vi "DepthCalibrationTable.vi"(11 "DS5CalibrationCoefficientsTable":u8[](array[numeric])=[21, 0, 0, 0, 3, 0, 25, 0, 240, 1, 0, 0, 0, 4, 0, 4, 169, 238, 63, 236, 156, 141, 55, 63, 113, 190, 162, 63, 135, 142, 252, 62, 9, 233, 5, 63, 31, 150, 10, 62, 55, 118, 207, 190, 113, 68, 102, 58, 249, 138, 146, 186, 37, 191, 183, 62, 140, 183, 56, 63, 9, 210, 163, 63, 166, 65, 2, 63, 224, 139, 1, 63, 100, 118, 2, 62, 234, 150, 203, 190, 17, 251, 198, 57, 162, 214, 21, 187, 174, 168, 180, 62, 233, 255, 127, 63, 123, 123, 122, 58, 169, 40, 178, 186, 91, 254, 122, 186, 231, 255, 127, 63, 249, 16, 188, 186, 151, 250, 177, 58, 148, 60, 188, 58, 223, 255, 127, 63, 253, 254, 127, 63, 187, 169, 2, 187, 133, 7, 170, 187, 170, 38, 3, 59, 205, 255, 127, 63, 195, 120, 187, 58, 120, 239, 169, 59, 115, 212, 188, 186, 13, 255, 127, 63, 197, 83, 91, 194, 1, 0, 0, 0, 0, 0, 0, 0, 0, 0, 0, 0, 0, 0, 0, 0, 0, 0, 0, 0, 0, 0, 0, 0, 0, 0, 0, 0, 0, 0, 0, 0, 0, 0, 0, 0, 0, 0, 0, 0, 0, 0, 0, 0, 0, 0, 0, 0, 0, 0, 0, 0, 0, 0, 0, 0, 0, 0, 0, 0, 0, 0, 0, 0, 0, 0, 0, 0, 0, 0, 0, 0, 0, 0, 0, 0, 0, 0, 0, 0, 0, 0, 0, 0, 0, 0, 0, 0, 0, 0, 0, 0, 27, 157, 178, 68, 27, 157, 178, 68, 254, 246, 109, 68, 45, 3, 11, 68, 207, 38, 110, 68, 207, 38, 110, 68, 169, 164, 30, 68, 145, 89, 185, 67, 138, 196, 30, 68, 138, 196, 30, 68, 225, 48, 158, 67, 23, 34, 119, 67, 138, 196, 30, 68, 138, 196, 30, 68, 225, 48, 210, 67, 23, 34, 119, 67, 207, 38, 238, 67, 207, 38, 238, 67, 169, 164, 158, 67, 145, 89, 57, 67, 138, 196, 158, 67, 138, 196, 158, 67, 225, 48, 82, 67, 23, 34, 247, 66, 138, 196, 158, 67, 138, 196, 158, 67, 225, 48, 30, 67, 23, 34, 247, 66, 27, 157, 178, 67, 27, 157, 178, 67, 254, 246, 109, 67, 45, 3, 11, 67, 115, 78, 132, 68, 115, 78, 132, 68, 17, 126, 30, 68, 190, 241, 205, 67, 27, 157, 50, 68, 27, 157, 50, 68, 254, 246, 237, 67, 45, 3, 139, 67, 0, 0, 0, 0, 0, 0, 0, 0, 0, 0, 0, 0, 0, 0, 0, 0, 0, 0, 0, 0, 0, 0, 0, 0, 0, 0, 0, 0, 0, 0, 0, 0, 0, 0, 0, 0, 0, 0, 0, 0, 0, 0, 0, 0, 0, 0, 0, 0, 0, 0, 0, 0, 0, 0, 0, 0, 0, 0, 0, 0, 0, 0, 0, 0, 0, 0, 0, 0, 0, 0, 0, 0, 0, 0, 0, 0, 0, 0, 0, 0, 0, 0, 0, 0, 0, 0, 0, 0, 0, 0, 0, 0, 0, 0, 0, 0, 0, 0, 0, 0, 105, 207, 27, 52, 0, 14, 0, 128, 67, 0, 58, 0, 92, 0, 80, 0, 114, 0, 111, 0, 103, 0, 114, 0, 97, 0, 109, 0, 32, 0, 70, 0, 105, 0, 108, 0, 101, 0, 115, 0, 92, 0, 78, 0, 97, 0, 116, 0, 105, 0, 111, 0, 110, 0, 97, 0, 108, 0, 32, 0, 73, 0, 110, 0, 115, 0, 116, 0, 114, 0, 117, 0, 109, 0, 101, 0, 110, 0, 116, 0, 115, 0, 92, 0, 76, 0, 97, 0, 98, 0, 86, 0, 73, 0, 69, 0, 87, 0, 32, 0, 50, 0, 48, 0, 49, 0, 54, 0, 92, 0, 76, 0, 97, 0, 98, 0, 86, 0, 73, 0, 69, 0, 87, 0, 46, 0, 101, 0, 120, 0, 101, 0, 0, 0, 114, 0, 101, 0, 92, 0, 112, 0, 110, 0, 103, 0, 46, 0, 108, 0, 108, 0, 98, 0, 0, 0, 0, 0, 0, 0, 0, 0, 0, 0, 0, 0, 0, 0, 0, 0, 0, 0, 0, 0, 0, 0, 0, 0, 0, 0, 0, 0, 0, 0, 0, 0, 0, 0, 0, 0, 0, 0, 0, 0, 0, 0, 0, 0, 0, 0, 0, 0, 0, 0, 0, 0, 0, 0, 0, 0, 0, 0, 0, 0, 0, 0, 0, 0, 0, 0, 0, 0, 0, 0, 0, 0, 0, 0, 0, 0, 0, 0, 0, 0, 0, 0, 0, 0, 0, 0, 0, 0, 0, 0, 0, 0, 0, 0, 0, 0, 0, 0, 0, 0, 0, 0, 0, 0, 0, 0, 0, 0, 0, 0, 0, 0, 0, 0, 0, 0, 0, 0, 0, 0, 0, 0, 0, 0, 0, 0, 0, 0, 0, 0, 0, 0, 0, 0, 0, 0, 0, 0, 0, 0, 0, 0, 0, 0, 0, 0, 0, 0, 0, 0, 0, 0, 0, 0, 0, 0, 0, 0, 0, 0, 0, 0, 0, 0, 0, 0, 0, 0, 0, 0, 0, 0, 0, 0, 0, 0, 0, 0, 0, 0, 0, 0, 0, 0, 0, 0, 0, 0, 0, 0, 0, 0, 0, 0, 0, 0, 0, 0, 0, 0, 0, 0, 0, 0, 0, 0, 0, 0, 0, 0, 0, 0, 0, 0, 0, 0, 0, 0, 0, 0, 0, 0, 0, 0, 0, 0, 0, 0, 0, 0, 0, 0, 0, 0, 0, 0, 0, 0, 0, 0, 0, 0, 0, 0, 0, 0, 0, 0, 0, 0, 0, 0, 0, 0, 0, 0, 0, 0, 0, 0, 0, 0, 0, 0, 0, 0, 0, 0, 0, 0, 0, 0, 0, 0, 0, 0, 0, 0, 0, 0, 0, 0, 0, 0, 0, 0, 0, 0, 0, 0, 0, 0, 0, 0, 0, 0, 0, 0, 0, 0, 0, 0, 0, 0, 0, 0, 0, 0, 0, 0, 0, 0, 0, 0, 0, 0, 0, 0, 0, 0, 0, 0, 0, 0, 0, 0, 0, 0, 0, 0, 0, 0, 0, 0, 0, 0, 0, 0, 0, 0, 0, 0, 0, 0, 0, 0, 0, 0, 0, 0] format="%x") -> (0 "table reserved 2":sgl[](array[numeric])=[714.4548, 714.4548, 475.92963, 278.0248], 1 "table reserved 1":sgl[](array[numeric])=[714.4548, 714.4548, 475.92963, 278.0248], 2 "New Calibration Parameters":T1={"fx"=0.71700454, "fy"=1.2714368, "px"=0.4932749, "py"=0.5230871, "k left"=[0.13533829, -0.40519878, 0.0008784002, -0.0011180333, 0.3588802], "fx2"=0.7215507, "fy2"=1.2798473, "py2"=0.5060406, "px2"=0.5088142, "k right"=[0.12740475, -0.39763576, 0.00037952562, -0.0022863527, 0.35284942], "RLeft"=[0.9999986, 0.0009555143, -0.001359244, -0.0009574645, 0.9999985, -0.001434832, 0.001357871, 0.0014361315, 0.99999803], "Rright"=[0.99998456, -0.0019937593, -0.0051888847, 0.002001206, 0.99999696, 0.0014302958, 0.0051860176, -0.0014406577, 0.9999855], "baseline"=-54.831806, "useBrownModel"=1, "1280x720"=[952.6064, 952.6064, 634.5728, 370.69974]}, 3 "Calibration table":T2={"version"=3, "table type"=60479, "table size"=496, "full version"=67109888, "crc32"=3963612841, "baseline"=-54.831806, "model"=1, "fx left"=917.7658, "fy left"=915.4345, "px left"=631.39185, "py left"=376.6227, "py right"=364.3492, "px right"=651.2822, "fy right"=921.49005, "fx right"=923.5849, "k left"=[0.13533829, -0.40519878, 0.0008784002, -0.0011180333, 0.3588802], "k right"=[0.12740475, -0.39763576, 0.00037952562, -0.0022863527, 0.35284942], "RLeft"=[0.9999986, 0.0009555143, -0.001359244, -0.0009574645, 0.9999985, -0.001434832, 0.001357871, 0.0014361315, 0.99999803], "Rright"=[0.99998456, -0.0019937593, -0.0051888847, 0.002001206, 0.99999696, 0.0014302958, 0.0051860176, -0.0014406577, 0.9999855], "uint8 reserved1"=[0, 0, 0, 0, 0, 0, 0, 0, 0, 0, 0, 0, 0, 0, 0, 0, 0, 0, 0, 0, 0, 0, 0, 0, 0, 0, 0, 0, 0, 0, 0, 0, 0, 0, 0, 0, 0, 0, 0, 0, 0, 0, 0, 0, 0, 0, 0, 0, 0, 0, 0, 0, 0, 0, 0, 0, 0, 0, 0, 0, 0, 0, 0, 0, 0, 0, 0, 0, 0, 0, 0, 0, 0, 0, 0, 0, 0, 0, 0, 0, 0, 0, 0, 0, 0, 0, 0, 0], "uint8 reserved2"=[0, 0, 0, 0, 0, 0, 0, 0, 0, 0, 0, 0, 0, 0, 0, 0, 0, 0, 0, 0, 0, 0, 0, 0, 0, 0, 0, 0, 0, 0, 0, 0, 0, 0, 0, 0, 0, 0, 0, 0, 0, 0, 0, 0, 0, 0, 0, 0, 0, 0, 0, 0, 0, 0, 0, 0, 0, 0, 0, 0, 0, 0, 0, 0], "1920x1080"=[1428.9095, 1428.9095, 951.85925, 556.0496], "1280x720"=[952.6064, 952.6064, 634.5728, 370.69974], "640x480"=[635.0709, 635.0709, 316.38187, 247.13316], "848x480"=[635.0709, 635.0709, 420.38187, 247.13316], "640x360"=[476.3032, 476.3032, 317.2864, 185.34987], "424x240"=[317.53546, 317.53546, 210.19093, 123.56658], "320x240"=[317.53546, 317.53546, 158.19093, 123.56658], "480x270"=[357.2274, 357.2274, 237.96481, 139.0124], "1280x800"=[1058.4515, 1058.4515, 633.9698, 411.8886], "960x540"=[714.4548, 714.4548, 475.92963, 278.0248], "Reserved1"=[714.4548, 714.4548, 475.92963, 278.0248], "Reserved 2"=[714.4548, 714.4548, 475.92963, 278.0248]} {"crc32" format="%x"})   [LabVIEW 2017, in "libRealSense3.lvlib"]
uses:
  libRealSense3.lvlib
panel:
  out "x+y":i32
  out "700":sgl[](array[numeric])=[1428.9095, 1428.9095, 951.85925, 556.0496]
  out "500":sgl[](array[numeric])=[1428.9095, 1428.9095, 951.85925, 556.0496]
  out "uint8 reserved2 2":u8[](array[numeric])
  out "Input size":i32
  out "size(s) 2":i32
  out "size(s)":i32
  out "size":i32
  out "subarray":u8[](array[numeric])=[156, 141, 55, 63, 113, 190, 162, 63, 135, 142, 252, 62, 9, 233, 5, 63, 31, 150, 10, 62, 55, 118, 207, 190, 113, 68, 102, 58, 249, 138, 146, 186, 37, 191, 183, 62] format="%x"
  out "Output array":u8[](array[numeric])=[3, 0, 25, 0, 240, 1, 0, 0, 0, 4, 0, 4, 169, 238, 63, 236, 156, 141, 55, 63, 113, 190, 162, 63, 135, 142, 252, 62, 9, 233, 5, 63, 31, 150, 10, 62, 55, 118, 207, 190, 113, 68, 102, 58, 249, 138, 146, 186, 37, 191, 183, 62, 140, 183, 56, 63, 9, 210, 163, 63, 166, 65, 2, 63, 224, 139, 1, 63, 100, 118, 2, 62, 234, 150, 203, 190, 17, 251, 198, 57, 162, 214, 21, 187, 174, 168, 180, 62, 233, 255, 127, 63, 123, 123, 122, 58, 169, 40, 178, 186, 91, 254, 122, 186, 231, 255, 127, 63, 249, 16, 188, 186, 151, 250, 177, 58, 148, 60, 188, 58, 223, 255, 127, 63, 253, 254, 127, 63, 187, 169, 2, 187, 133, 7, 170, 187, 170, 38, 3, 59, 205, 255, 127, 63, 195, 120, 187, 58, 120, 239, 169, 59, 115, 212, 188, 186, 13, 255, 127, 63, 197, 83, 91, 194, 1, 0, 0, 0, 0, 0, 0, 0, 0, 0, 0, 0, 0, 0, 0, 0, 0, 0, 0, 0, 0, 0, 0, 0, 0, 0, 0, 0, 0, 0, 0, 0, 0, 0, 0, 0, 0, 0, 0, 0, 0, 0, 0, 0, 0, 0, 0, 0, 0, 0, 0, 0, 0, 0, 0, 0, 0, 0, 0, 0, 0, 0, 0, 0, 0, 0, 0, 0, 0, 0, 0, 0, 0, 0, 0, 0, 0, 0, 0, 0, 0, 0, 0, 0, 0, 0, 0, 0, 0, 0, 0, 0, 27, 157, 178, 68, 27, 157, 178, 68, 254, 246, 109, 68, 45, 3, 11, 68, 207, 38, 110, 68, 207, 38, 110, 68, 169, 164, 30, 68, 145, 89, 185, 67, 138, 196, 30, 68, 138, 196, 30, 68, 225, 48, 158, 67, 23, 34, 119, 67, 138, 196, 30, 68, 138, 196, 30, 68, 225, 48, 210, 67, 23, 34, 119, 67, 207, 38, 238, 67, 207, 38, 238, 67, 169, 164, 158, 67, 145, 89, 57, 67, 138, 196, 158, 67, 138, 196, 158, 67, 225, 48, 82, 67, 23, 34, 247, 66, 138, 196, 158, 67, 138, 196, 158, 67, 225, 48, 30, 67, 23, 34, 247, 66, 27, 157, 178, 67, 27, 157, 178, 67, 254, 246, 109, 67, 45, 3, 11, 67, 115, 78, 132, 68, 115, 78, 132, 68, 17, 126, 30, 68, 190, 241, 205, 67, 27, 157, 50, 68, 27, 157, 50, 68, 254, 246, 237, 67, 45, 3, 139, 67] format="%x"
  out "Baseline":u8[](array[numeric])=[194, 91, 83, 197]
  out "reversed array":u8[](array[numeric])=[194, 91, 83, 197]
  out "960x540":sgl[](array[numeric])=[714.4548, 714.4548, 475.92963, 278.0248]
  out "1280x800":sgl[](array[numeric])=[1058.4515, 1058.4515, 633.9698, 411.8886]
  out "480x270":sgl[](array[numeric])=[357.2274, 357.2274, 237.96481, 139.0124]
  out "320x240":sgl[](array[numeric])=[317.53546, 317.53546, 158.19093, 123.56658]
  out "424x240":sgl[](array[numeric])=[317.53546, 317.53546, 210.19093, 123.56658]
  out "640x360":sgl[](array[numeric])=[476.3032, 476.3032, 317.2864, 185.34987]
  out "848x480":sgl[](array[numeric])=[635.0709, 635.0709, 420.38187, 247.13316]
  out "640x480":sgl[](array[numeric])=[635.0709, 635.0709, 316.38187, 247.13316]
  out "1280x720":sgl[](array[numeric])=[952.6064, 952.6064, 634.5728, 370.69974]
  out "1920x1080":sgl[](array[numeric])=[1428.9095, 1428.9095, 951.85925, 556.0496]
  out "uint8 reserved2":u8[](array[numeric])
  out "uint8 reserved1":u8[](array[numeric])
  out "model":u32=1
  out "baseline":sgl=-54.831806
  out "Rright":sgl[](array[numeric])=[0.99998456, -0.0019937593, -0.0051888847, 0.002001206, 0.99999696, 0.0014302958, 0.0051860176, -0.0014406577, 0.9999855]
  out "RLeft":sgl[](array[numeric])=[0.9999986, 0.0009555143, -0.001359244, -0.0009574645, 0.9999985, -0.001434832, 0.001357871, 0.0014361315, 0.99999803]
  out "crc32":u32=3963612841
  out "full version":u32=67109888
  out "table size":u32=496
  out "table type":u16=25
  out "version":u16=3
  out "fx2":sgl=0.7215507
  out "fy2":sgl=1.2798473
  out "px2":sgl=0.5088142
  out "py2":sgl=0.5060406
  out "k right":sgl[](array[numeric])=[0.12740475, -0.39763576, 0.00037952562, -0.0022863527, 0.35284942]
  out "k left":sgl[](array[numeric])=[0.13533829, -0.40519878, 0.0008784002, -0.0011180333, 0.3588802]
  out "py":sgl=0.5230871
  out "px":sgl=0.4932749
  out "fy":sgl=1.2714368
  out "fx":sgl=0.71700454
  # "this is to get coefficents"
  # "//! DS5 calibration coefficients table. Table ID is 0x19.\nstruct DS5CalibrationCoefficientsTable\n{\n\tDS5CalibrationTableHeader header;       //!< Header\n\tDS5CalibrationCoefficients coeffs;      //!< Coefficients\n\tDS5CoeffsMode  modes[12];               //!< Rectified camera parameters. Each entry in the table corresponds to a resolution\n\tuint8_t  reserved2[64];                 //!< Reserved\n};"
  # "Use this one to set through intermediate"
  # "//! Structure used to update the calibration during live streaming using the CALIBRECALC command\nstruct DS5CalibrationCoefficientsUpdateParam\n{\n\tDS5CalibrationCoefficients coeffs;      //!< Coefficients\n\tDS5CoeffsMode mode;                     //!< Rectified camera parameters for the current resolution\n};"
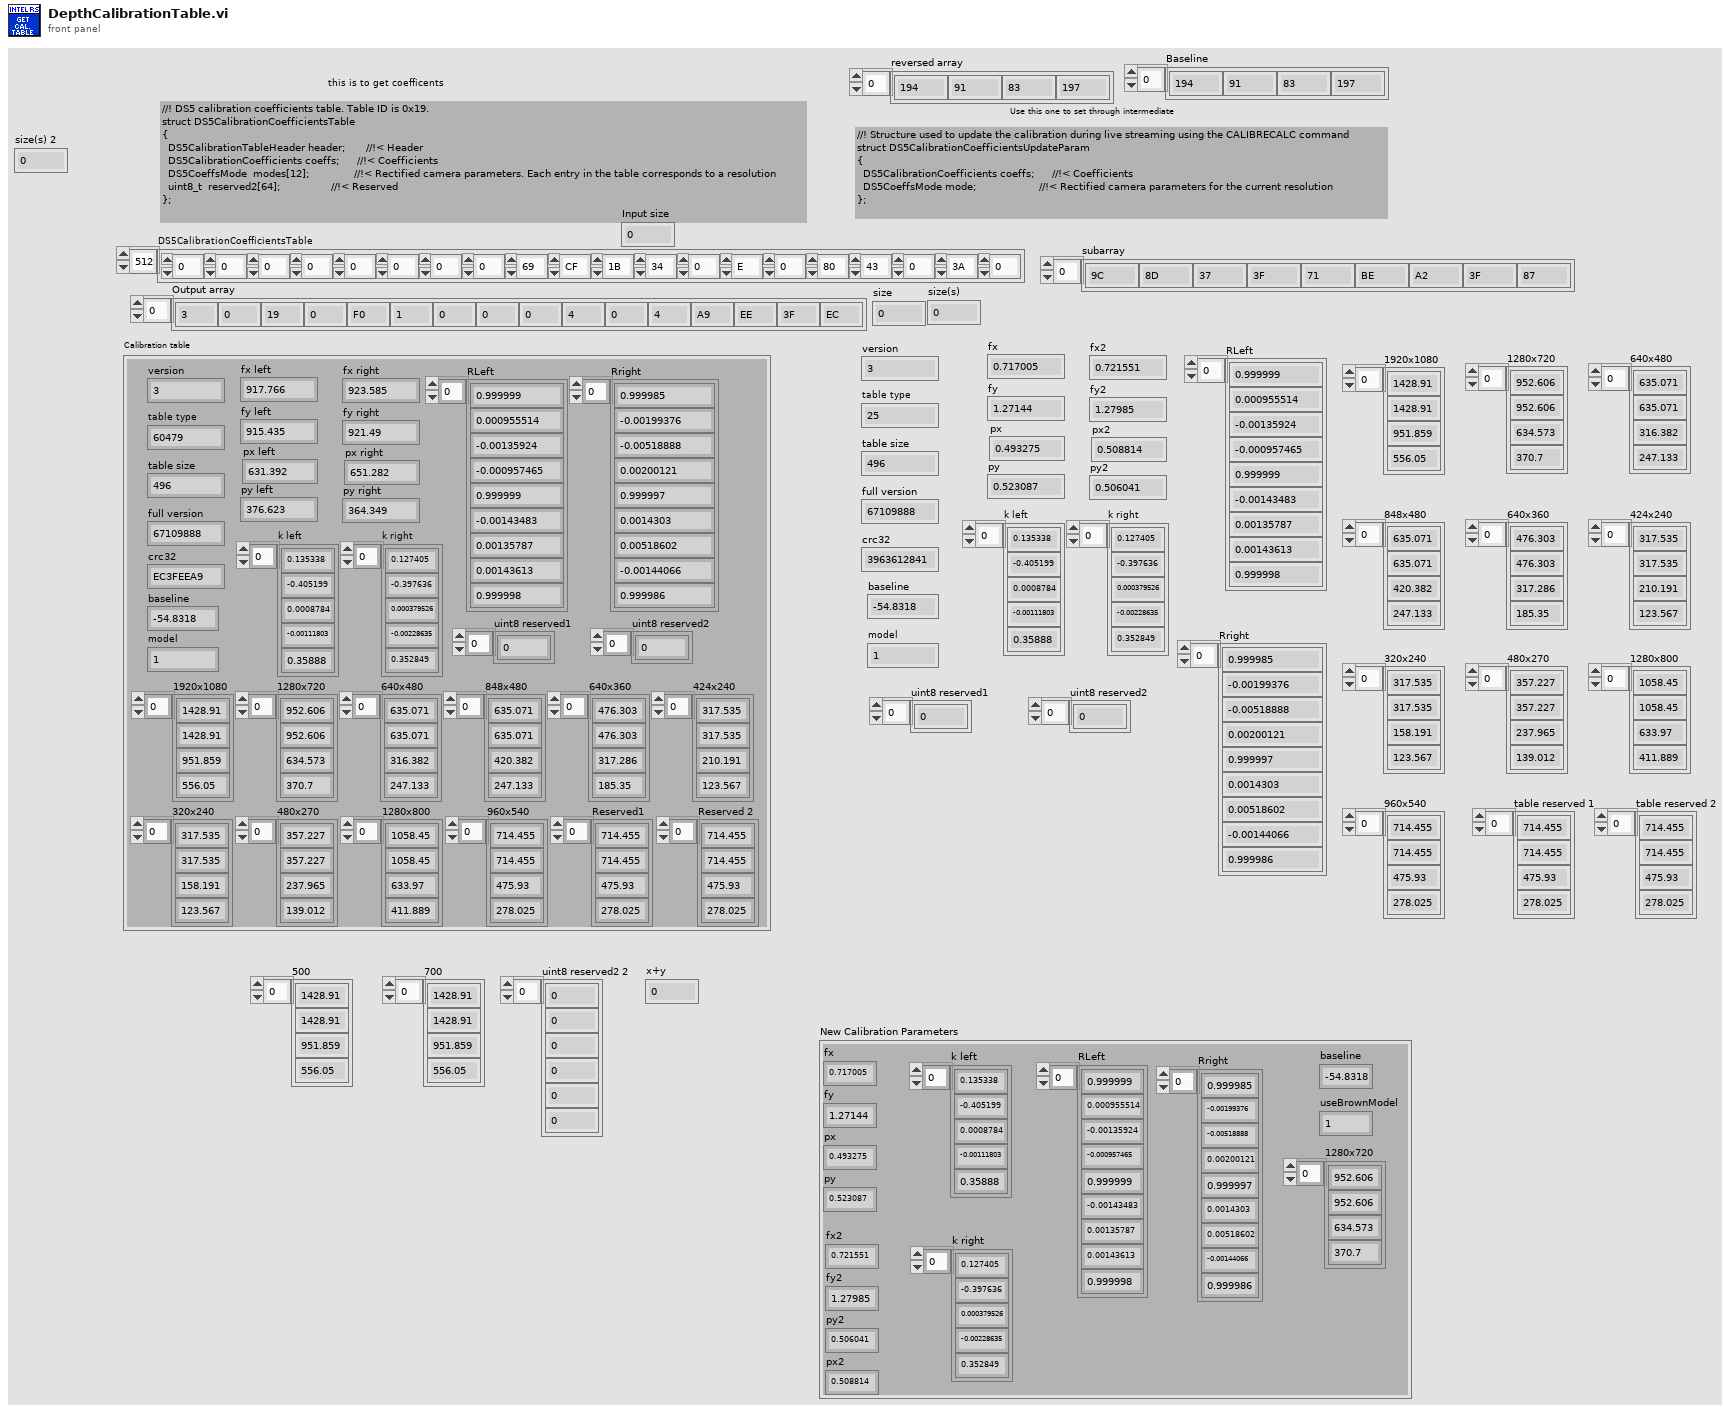
[diagram p1: front panel]
types:
  T1 = cluster{"fx":sgl, "fy":sgl, "px":sgl, "py":sgl, "k left":sgl[], "fx2":sgl, "fy2":sgl, "py2":sgl, "px2":sgl, "k right":sgl[], "RLeft":sgl[], "Rright":sgl[], "baseline":sgl, "useBrownModel":u32, "1280x720":sgl[]}
  T2 = cluster{"version":u16, "table type":u16, "table size":u32, "full version":u32, "crc32":u32, "baseline":sgl, "model":u32, "fx left":sgl, "fy left":sgl, "px left":sgl, "py left":sgl, "py right":sgl, "px right":sgl, "fy right":sgl, "fx right":sgl, "k left":sgl[], "k right":sgl[], "RLeft":sgl[], "Rright":sgl[], "uint8 reserved1":u8[], "uint8 reserved2":u8[], "1920x1080":sgl[], "1280x720":sgl[], "640x480":sgl[], "848x480":sgl[], "640x360":sgl[], "424x240":sgl[], "320x240":sgl[], "480x270":sgl[], "1280x800":sgl[], "960x540":sgl[], "Reserved1":sgl[], "Reserved 2":sgl[]}
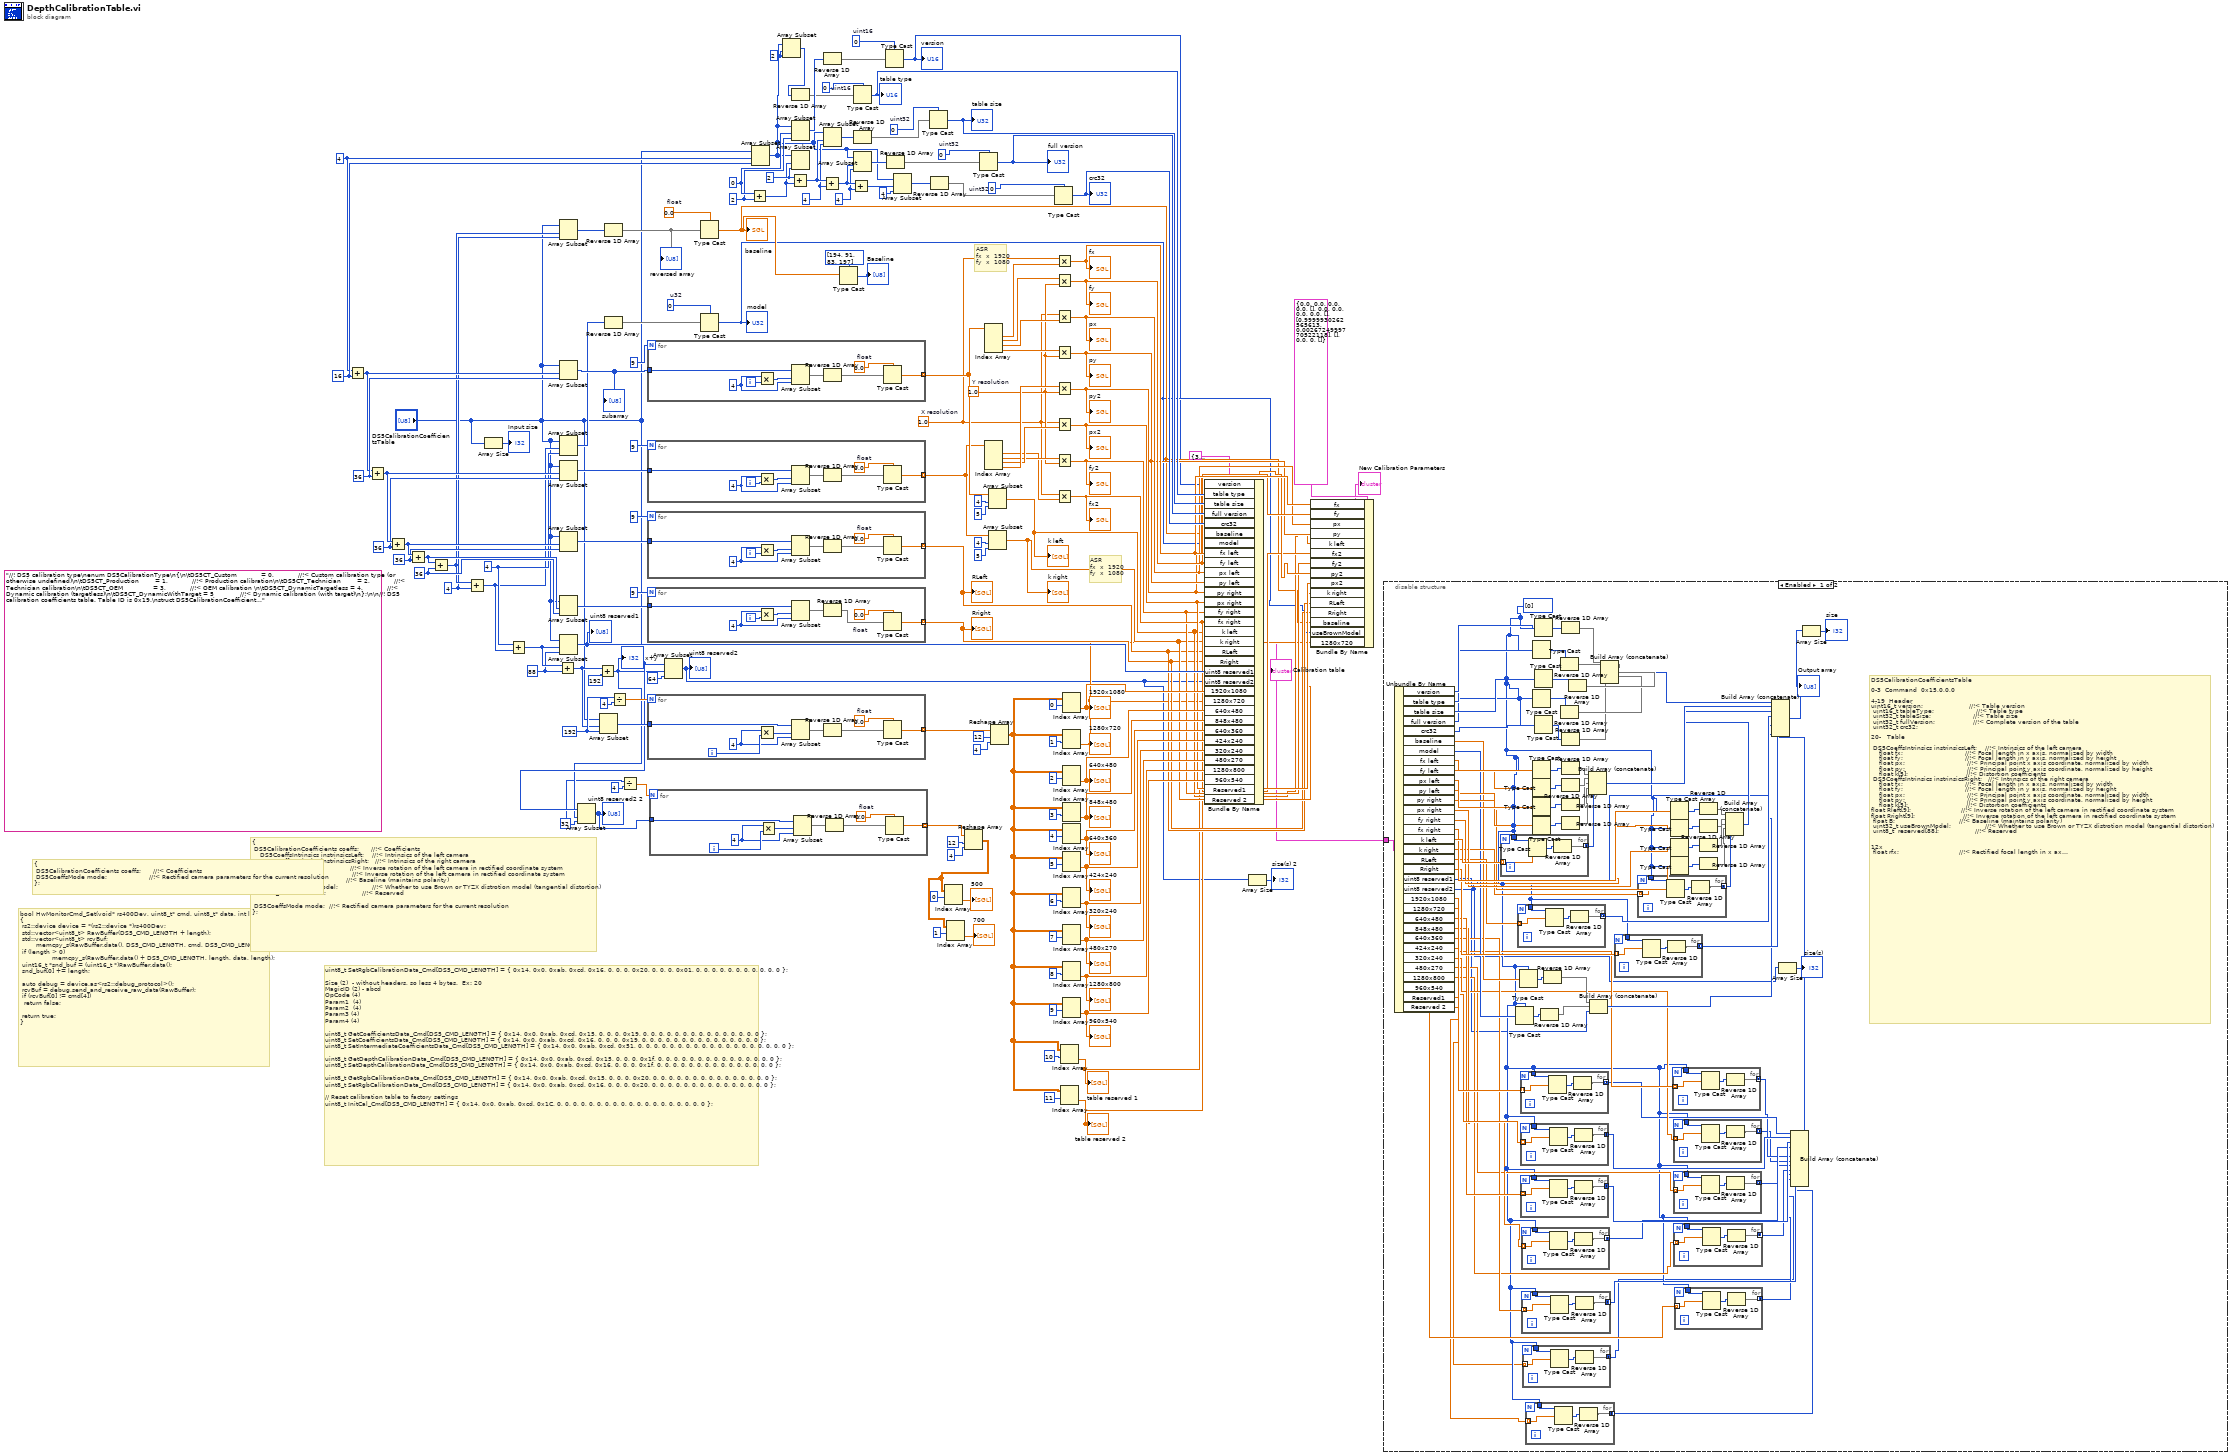
[diagram p0: block diagram]
diagram:
  w10 = 32 ("length")
  w27 = 2 ("length")
  w131 = sgl 1.0  # Y resolution
  w130 = sgl 1.0  # X resolution
  (unwired) "//! DS5 calibration type\nenum DS5CalibrationType\n{\n\tDS5CT_Custom            = 0,            //!< Custom calibration type (or otherwise undefined)\n\tDS5CT_Production        = 1,            //!< Production calibration\n\tDS5CT_Technician        = 2,            //!< Technician calibration\n\tDS5CT_OEM               = 3,            //!< OEM calibration \n\tDS5CT_DynamicTargetless = 4,            //!< Dynamic calibration (targetless)\n\tDS5CT_DynamicWithTarget = 5             //!< Dynamic calibration (with target)\n};\n\n//! DS5 calibration coefficients table. Table ID is 0x19.\nstruct DS5CalibrationCoefficientsTable\n{\n\tDS5CalibrationTableHeader header;       //!< Header\n\tDS5CalibrationCoefficients coeffs;      //!< Coefficients\n\tDS5CoeffsMode  modes[12];               //!< Rectified camera parameters. Each entry in the table corresponds to a resolution\n\tuint8_t  reserved2[64];                 //!< Reserved\n};\n\nstruct DS5CalibrationTableHeader\n{\n\tuint16_t version;                       //!< Table version\n\tuint16_t tableType;                     //!< Table type\n\tuint32_t tableSize;                     //!< Table size \n\tuint32_t fullVersion;                   //!< Complete version of the table\n\tuint32_t crc32;                         //!< CRC32 of the content\n};\n\nstruct DS5CalibrationCoefficients\n{\n\tDS5CoeffsIntrinsics instrinsicsLeft;    //!< Intrinsics of the left camera\n\tDS5CoeffsIntrinsics instrinsicsRight;   //!< Intrinsics of the right camera\n\tfloat Rleft[9];                         //!< Inverse rotation of the left camera in rectified coordinate system\n\tfloat Rright[9];                        //!< Inverse rotation of the left camera in rectified coordinate system\n\tfloat B;                                //!< Baseline (maintains polarity)\n\tuint32_t useBrownModel;                 //!< Whether to use Brown or TYZX distrotion model (tangential distortion)\n\tuint8_t  reserved[88];                  //!< Reserved\n};\n\nstruct DS5CoeffsMode\n{\n\tfloat rfx;                              //!< Rectified focal length in x axis\n\tfloat rfy;                              //!< Rectified focal length in y axis\n\tfloat rpx;                              //!< Rectified principal point x axis coordinate\n\tfloat rpy;                              //!< Rectified principal point y axis coordinate\n};\n\nstruct DS5CoeffsIntrinsics\n{\n\tfloat fx;                               //!< Focal length in x axis, normalized by width\n\tfloat fy;                               //!< Focal length in y axis, normalized by height\n\tfloat px;                               //!< Principal point x axis coordinate, normalized by width\n\tfloat py;                               //!< Principal point y axis coordinate, normalized by height\n\tfloat k[5];                             //!< Distortion coefficients\n};\n\n/** \\brief Distortion model: defines how pixel coordinates should be mapped to sensor coordinates. */\ntypedef enum rs2_distortion\n{\n    RS2_DISTORTION_NONE                  , /**< Rectilinear images. No distortion compensation required. */\n    RS2_DISTORTION_MODIFIED_BROWN_CONRADY, /**< Equivalent to Brown-Conrady distortion, except that tangential distortion is applied to radially distorted points */\n    RS2_DISTORTION_INVERSE_BROWN_CONRADY , /**< Equivalent to Brown-Conrady distortion, except undistorts image instead of distorting it */\n    RS2_DISTORTION_FTHETA                , /**< F-Theta fish-eye distortion model */\n    RS2_DISTORTION_BROWN_CONRADY         , /**< Unmodified Brown-Conrady distortion model */\n    RS2_DISTORTION_COUNT                 , /**< Number of enumeration values. Not a valid input: intended to be used in for-loops. */\n} rs2_distortion;\n\n//! DS5 recitifed resolution index\nenum DS5CoeffsModeIndex\n{\n\tDS5M_1920_1080 = 0,                     //!< 1920x1080 rectified resolution (R8L8 only)\n\tDS5M_1280_720  = 1,                     //!< 1280x720 rectified resolution\n\tDS5M_640_480   = 2,                     //!< 640x480 rectified resolution\n\tDS5M_848_480   = 3,                     //!< 848x480 rectified resolution\n\tDS5M_640_360   = 4,                     //!< 640x360 rectified resolution\n\tDS5M_424_240   = 5,                     //!< 424x240 rectified resolution\n\tDS5M_320_240   = 6,                     //!< 320x240 rectified resolution\n\tDS5M_480_270   = 7,                     //!< 480x270 rectified resolution\n\tDS5M_1280_800  = 8,                     //!< 1280x800 rectified resolution (R8L8 only)\n\tDS5M_960_540   = 9                      //!< 960x540 rectified resolution\n};"
  w74 = 192 ("length")
  w82 = 88 ("length")
  w89 = u32 0  # u32
  w85 = 4 ("length")
  w92 = sgl 0.0  # float
  w86 = 4 ("length")
  w97 = 36 ("length")
  w100 = 36 ("length")
  w104 = u32 0  # uint32
  w111 = u32 0  # uint32
  w105 = 4 ("index")
  w116 = u32 0  # uint32
  w119 = u16 0  # uint16
  w121 = u16 0  # uint16
  w113 = 4 ("index")
  w125 = 2 ("index")
  w126 = 2 ("index")
  w127 = 0 ("index")
  w128 = 36 ("length")
  w144 = 4 ("index")
  w146 = 16 ("length")
  w150 = 36 ("length")
  # "{\n\tDS5CalibrationCoefficients coeffs;      //!< Coefficients\n\t   DS5CoeffsIntrinsics instrinsicsLeft;    //!< Intrinsics of the left camera\n\t   DS5CoeffsIntrinsics instrinsicsRight;   //!< Intrinsics of the right camera\n\t   float Rleft[9];                         //!< Inverse rotation of the left camera in rectified coordinate system\n\t   float Rright[9];                        //!< Inverse rotation of the left camera in rectified coordinate system\n\t   float B;                                //!< Baseline (maintains polarity)\n\t   uint32_t useBrownModel;                 //!< Whether to use Brown or TYZX distrotion model (tangential distortion)\n\t   uint8_t  reserved[88];                  //!< Reserved\n\t\n\tDS5CoeffsMode mode;  //!< Rectified camera parameters for the current resolution \n};"
  # "uint8_t SetRgbCalibrationData_Cmd[DS5_CMD_LENGTH] = { 0x14, 0x0, 0xab, 0xcd, 0x16, 0, 0, 0, 0x20, 0, 0, 0, 0x01, 0, 0, 0, 0, 0, 0, 0, 0, 0, 0, 0 };\n\nSize (2)  - without headers, so less 4 bytes.  Ex: 20\nMagicID (2) - abcd\nOpCode (4)\nParam1  (4)\nParam2  (4)\nParam3 (4)\nParam4 (4)\n\nuint8_t GetCoefficientsData_Cmd[DS5_CMD_LENGTH] = { 0x14, 0x0, 0xab, 0xcd, 0x15, 0, 0, 0, 0x19, 0, 0, 0, 0, 0, 0, 0, 0, 0, 0, 0, 0, 0, 0, 0 };\nuint8_t SetCoefficientsData_Cmd[DS5_CMD_LENGTH] = { 0x14, 0x0, 0xab, 0xcd, 0x16, 0, 0, 0, 0x19, 0, 0, 0, 0, 0, 0, 0, 0, 0, 0, 0, 0, 0, 0, 0 };\nuint8_t SetIntermediateCoefficientsData_Cmd[DS5_CMD_LENGTH] = { 0x14, 0x0, 0xab, 0xcd, 0x51, 0, 0, 0, 0, 0, 0, 0, 0, 0, 0, 0, 0, 0, 0, 0, 0, 0, 0, 0 };\n\nuint8_t GetDepthCalibrationData_Cmd[DS5_CMD_LENGTH] = { 0x14, 0x0, 0xab, 0xcd, 0x15, 0, 0, 0, 0x1f, 0, 0, 0, 0, 0, 0, 0, 0, 0, 0, 0, 0, 0, 0, 0 };\nuint8_t SetDepthCalibrationData_Cmd[DS5_CMD_LENGTH] = { 0x14, 0x0, 0xab, 0xcd, 0x16, 0, 0, 0, 0x1f, 0, 0, 0, 0, 0, 0, 0, 0, 0, 0, 0, 0, 0, 0, 0 };\n\nuint8_t GetRgbCalibrationData_Cmd[DS5_CMD_LENGTH] = { 0x14, 0x0, 0xab, 0xcd, 0x15, 0, 0, 0, 0x20, 0, 0, 0, 0, 0, 0, 0, 0, 0, 0, 0, 0, 0, 0, 0 };\nuint8_t SetRgbCalibrationData_Cmd[DS5_CMD_LENGTH] = { 0x14, 0x0, 0xab, 0xcd, 0x16, 0, 0, 0, 0x20, 0, 0, 0, 0, 0, 0, 0, 0, 0, 0, 0, 0, 0, 0, 0 };\n\n// Reset calibration table to factory settings\nuint8_t InitCal_Cmd[DS5_CMD_LENGTH] = { 0x14, 0x0, 0xab, 0xcd, 0x1C, 0, 0, 0, 0, 0, 0, 0, 0, 0, 0, 0, 0, 0, 0, 0, 0, 0, 0, 0 };"
  # "{\n\tDS5CalibrationCoefficients coeffs;      //!< Coefficients\n\tDS5CoeffsMode mode;                     //!< Rectified camera parameters for the current resolution\n};"
  # "bool HwMonitorCmd_Set(void* rs400Dev, uint8_t* cmd, uint8_t* data, int length)\n{\n\trs2::device device = *(rs2::device *)rs400Dev;\n\tstd::vector<uint8_t> RawBuffer(DS5_CMD_LENGTH + length);\n\tstd::vector<uint8_t> rcvBuf;\n        memcpy_s(RawBuffer.data(), DS5_CMD_LENGTH, cmd, DS5_CMD_LENGTH);\n\tif (length > 0)\n                memcpy_s(RawBuffer.data() + DS5_CMD_LENGTH, length, data, length);\n\tuint16_t *snd_buf = (uint16_t *)RawBuffer.data();\n\tsnd_buf[0] += length;\n\n\tauto debug = device.as<rs2::debug_protocol>();\n\trcvBuf = debug.send_and_receive_raw_data(RawBuffer);\n\tif (rcvBuf[0] != cmd[4])\n\t\treturn false;\n\n\treturn true;\n}"
  # "ASR\nfx  x  1920\nfy  x  1080"
  # "ASR\nfx  x  1920\nfy  x  1080"
  n1 = Add(x=w144, y=w146) -> (x+y=w145:i32)
  n2 = Add(x=w145, y=w150) -> (x+y=w129:i32)
  n3 = Add(x=w129, y=w128) -> (x+y=w101:i32)
  n4 = Add(x=w101, y=w100) -> (x+y=w94:i32)
  n5 = Add(x=w94, y=w97) -> (x+y=w87:i32)
  n6 = Add(x=w87, y=w86) -> (x+y=w84:i32)
  n7 = Array Size(array="DS5CalibrationCoefficientsTable") -> (size(s)=→"Input size":i32)
  n8 = Add(x=w85, y=w84) -> (x+y=w83:i32)
  n9 = Add(x=w83, y=w82) -> (x+y=w16:i32)
  n10 = Array Subset(array="DS5CalibrationCoefficientsTable", index=w87, length=w86) -> (w91:u8[])
  n11 = Array Subset(array="DS5CalibrationCoefficientsTable", index=w145, length=w150) -> (w151:u8[])
  "subarray" <- w151
  n12 = Array Subset(array="DS5CalibrationCoefficientsTable", index=w84, length=w85) -> (w90:u8[])
  n13 = Array Subset(array="DS5CalibrationCoefficientsTable", index=w129, length=w128) -> (w132:u8[])
  n14 = Array Subset(array="DS5CalibrationCoefficientsTable", index=w101, length=w100) -> (w103:u8[])
  n15 = Array Subset(array="DS5CalibrationCoefficientsTable", index=w94, length=w97) -> (w95:u8[])
  n16 = Array Subset(array="DS5CalibrationCoefficientsTable", index=w83, length=w82) -> (w59:u8[])
  "uint8 reserved1" <- w59
  n17 = Add(x=w16, y=192) -> (x+y=w13:i32)
  "x+y" <- w13
  n18 = Array Subset(array="DS5CalibrationCoefficientsTable", index=w13, length=w10) -> (w12:u8[])
  "uint8 reserved2 2" <- w12
  n19 = Array Subset(array="DS5CalibrationCoefficientsTable", index=w16, length=w74) -> (w81:u8[])
  n20 = Reverse 1D Array(array=w91) -> (reversed array=w93:u8[])
  "reversed array" <- w93
  n21 = Reverse 1D Array(array=w90) -> (reversed array=w88:u8[])
  n22 = Divide(x=w74, y=4) -> (x/y=w80:dbl)
  n23 = Divide(x=w10, y=4) -> (x/y=w9:dbl)
  n24 = for {
    N: 9 -> [_]
    tunnel: w151 -> [w158]
    tunnel: [w152] -> w148 mode=indexing
    i -> [w155]
    w154 = 4 ("length")
    w159 = sgl 0.0  # float
    n25 = Multiply(x=w154, y=w155) -> (x*y=w153:i32)
    n26 = Array Subset(array=w158, index=w153, length=w154) -> (w156:u8[])
    n27 = Reverse 1D Array(array=w156) -> (reversed array=w157:u8[])
    n28 = Type Cast(type=w159, x=w157) -> (*(type *) &x=w152:sgl)
  }
  n29 = for {
    N: 9 -> [_]
    tunnel: w132 -> [w166]
    tunnel: [w160] -> w134 mode=indexing
    i -> [w163]
    w162 = 4 ("length")
    w167 = sgl 0.0  # float
    n30 = Multiply(x=w162, y=w163) -> (x*y=w161:i32)
    n31 = Array Subset(array=w166, index=w161, length=w162) -> (w164:u8[])
    n32 = Reverse 1D Array(array=w164) -> (reversed array=w165:u8[])
    n33 = Type Cast(type=w167, x=w165) -> (*(type *) &x=w160:sgl)
  }
  n34 = for {
    N: 9 -> [_]
    tunnel: w103 -> [w174]
    tunnel: [w168] -> w35 mode=indexing
    i -> [w171]
    w170 = 4 ("length")
    w175 = sgl 0.0  # float
    n35 = Multiply(x=w170, y=w171) -> (x*y=w169:i32)
    n36 = Array Subset(array=w174, index=w169, length=w170) -> (w172:u8[])
    n37 = Reverse 1D Array(array=w172) -> (reversed array=w173:u8[])
    n38 = Type Cast(type=w175, x=w173) -> (*(type *) &x=w168:sgl)
  }
  "RLeft" <- w35
  n39 = for {
    N: 9 -> [_]
    tunnel: w95 -> [w182]
    tunnel: [w176] -> w34 mode=indexing
    i -> [w179]
    w178 = 4 ("length")
    w183 = sgl 0.0  # float
    n40 = Multiply(x=w178, y=w179) -> (x*y=w177:i32)
    n41 = Array Subset(array=w182, index=w177, length=w178) -> (w180:u8[])
    n42 = Reverse 1D Array(array=w180) -> (reversed array=w181:u8[])
    n43 = Type Cast(type=w183, x=w181) -> (*(type *) &x=w176:sgl)
  }
  "Rright" <- w34
  n44 = for {
    N: w80 -> [_]
    tunnel: w81 -> [w190]
    tunnel: [w184] -> w78 mode=indexing
    i -> [w187]
    w186 = 4 ("length")
    w191 = sgl 0.0  # float
    n45 = Multiply(x=w186, y=w187) -> (x*y=w185:i32)
    n46 = Array Subset(array=w190, index=w185, length=w186) -> (w188:u8[])
    n47 = Reverse 1D Array(array=w188) -> (reversed array=w189:u8[])
    n48 = Type Cast(type=w191, x=w189) -> (*(type *) &x=w184:sgl)
  }
  n49 = for {
    N: w9 -> [_]
    tunnel: w12 -> [w198]
    tunnel: [w192] -> w6 mode=indexing
    i -> [w195]
    w194 = 4 ("length")
    w199 = sgl 0.0  # float
    n50 = Multiply(x=w194, y=w195) -> (x*y=w193:i32)
    n51 = Array Subset(array=w198, index=w193, length=w194) -> (w196:u8[])
    n52 = Reverse 1D Array(array=w196) -> (reversed array=w197:u8[])
    n53 = Type Cast(type=w199, x=w197) -> (*(type *) &x=w192:sgl)
  }
  n54 = Array Subset(array="DS5CalibrationCoefficientsTable", index=w13, length=64) -> (w18:u8[])
  "uint8 reserved2" <- w18
  n55 = Type Cast(type=w92, x=w93) -> (*(type *) &x=w33:sgl)
  "baseline" <- w33
  n56 = Type Cast(type=w89, x=w88) -> (*(type *) &x=w32:u32)
  "model" <- w32
  n57 = Add(x=w127, y=w126) -> (x+y=w124:i32)
  n58 = Array Subset(array="DS5CalibrationCoefficientsTable", index=w144, length=w146) -> (w29:u8[])
  n59 = Array Subset(array=w29, index=w27, length=w27) -> (w28:u8[])
  n60 = Add(x=w125, y=w124) -> (x+y=w114:i32)
  n61 = Reverse 1D Array(array=w28) -> (reversed array=w120:u8[])
  n62 = Array Subset(array=w29, index=w127, length=w126) -> (w122:u8[])
  n63 = Array Subset(array=w29, index=w124, length=w125) -> ()  [unwired: 1 out]
  n64 = Add(x=w114, y=w113) -> (x+y=w106:i32)
  n65 = Reverse 1D Array(array=w122) -> (reversed array=w123:u8[])
  n66 = Array Subset(array=w29, index=w114, length=w113) -> (w117:u8[])
  n67 = Type Cast(type=u8[] [194, 91, 83, 197] ("reversed array"), x=w33) -> (*(type *) &x=→"Baseline":u8[])
  n68 = Add(x=w106, y=w105) -> (x+y=w109:i32)
  n69 = Type Cast(type=w119, x=w120) -> (*(type *) &x=w63:u16)
  "table type" <- w63
  n70 = Reverse 1D Array(array=w117) -> (reversed array=w118:u8[])
  n71 = Array Subset(array=w29, index=w106, length=w105) -> (w115:u8[])
  n72 = Type Cast(type=w121, x=w123) -> (*(type *) &x=w30:u16)
  "version" <- w30
  n73 = Reverse 1D Array(array=w115) -> (reversed array=w112:u8[])
  n74 = Array Subset(array=w29, index=w109, length=4 ("index")) -> (w107:u8[])
  n75 = Type Cast(type=w116, x=w118) -> (*(type *) &x=w62:u32)
  "table size" <- w62
  n76 = Reverse 1D Array(array=w107) -> (reversed array=w110:u8[])
  n77 = Reshape Array(w6, 12 ("dimension size"), 4 ("dimension size")) -> (w1:sgl[][])
  n78 = Index Array(array=w1, index (row)=0) -> (element=→"500":sgl[])  [unwired: 1 in]
  n79 = Index Array(array=w1, index (row)=1) -> (element=→"700":sgl[])  [unwired: 1 in]
  n80 = Type Cast(type=w111, x=w112) -> (*(type *) &x=w61:u32)
  "full version" <- w61
  n81 = Index Array(array=w148) -> (element #1=w143:sgl, element #2=w142:sgl, element #3=w141:sgl, element #4=w140:sgl)  [unwired: 4 in]
  n82 = Index Array(array=w134) -> (element #1=w136:sgl, element #2=w137:sgl, element #3=w138:sgl, element #4=w139:sgl)  [unwired: 4 in]
  n83 = Array Subset(array=w148, index=4, length=5) -> (w37:sgl[])
  "k left" <- w37
  n84 = Array Subset(array=w134, index=4, length=5) -> (w36:sgl[])
  "k right" <- w36
  n85 = Reshape Array(w78, 12 ("dimension size"), 4 ("dimension size")) -> (w25:sgl[][])
  n86 = Type Cast(type=w104, x=w110) -> (*(type *) &x=w60:u32)
  "crc32" <- w60
  n87 = Multiply(x=w130, y=w143) -> (x*y=w45:sgl)
  "fx" <- w45
  n88 = Multiply(x=w142, y=w131) -> (x*y=w44:sgl)
  "fy" <- w44
  n89 = Multiply(x=w130, y=w141) -> (x*y=w43:sgl)
  "px" <- w43
  n90 = Multiply(x=w140, y=w131) -> (x*y=w42:sgl)
  "py" <- w42
  n91 = Multiply(x=w139, y=w131) -> (x*y=w41:sgl)
  "py2" <- w41
  n92 = Multiply(x=w130, y=w138) -> (x*y=w40:sgl)
  "px2" <- w40
  n93 = Multiply(x=w137, y=w131) -> (x*y=w38:sgl)
  "fy2" <- w38
  n94 = Multiply(x=w130, y=w136) -> (x*y=w39:sgl)
  "fx2" <- w39
  n95 = Index Array(array=w25, index (row)=10) -> (element=w21:sgl[])  [unwired: 1 in]
  "table reserved 1" <- w21
  n96 = Index Array(array=w25, index (row)=11) -> (element=w20:sgl[])  [unwired: 1 in]
  "table reserved 2" <- w20
  n97 = Index Array(array=w25, index (row)=0) -> (element=w58:sgl[])  [unwired: 1 in]
  "1920x1080" <- w58
  n98 = Index Array(array=w25, index (row)=1) -> (element=w31:sgl[])  [unwired: 1 in]
  "1280x720" <- w31
  n99 = Index Array(array=w25, index (row)=2) -> (element=w57:sgl[])  [unwired: 1 in]
  "640x480" <- w57
  n100 = Index Array(array=w25, index (row)=3) -> (element=w56:sgl[])  [unwired: 1 in]
  "848x480" <- w56
  n101 = Index Array(array=w25, index (row)=4) -> (element=w55:sgl[])  [unwired: 1 in]
  "640x360" <- w55
  n102 = Index Array(array=w25, index (row)=5) -> (element=w54:sgl[])  [unwired: 1 in]
  "424x240" <- w54
  n103 = Index Array(array=w25, index (row)=6) -> (element=w53:sgl[])  [unwired: 1 in]
  "320x240" <- w53
  n104 = Index Array(array=w25, index (row)=7) -> (element=w52:sgl[])  [unwired: 1 in]
  "480x270" <- w52
  n105 = Index Array(array=w25, index (row)=8) -> (element=w51:sgl[])  [unwired: 1 in]
  "1280x800" <- w51
  n106 = Index Array(array=w25, index (row)=9) -> (element=w50:sgl[])  [unwired: 1 in]
  "960x540" <- w50
  n107 = Bundle By Name(cluster=T2 {"version"=3, "table type"=60479, "table size"=496, "full version"=67109888, "crc32"=3963612841, "baseline"=-54.831806, "model"=1, "fx left"=917.7658, "fy left"=915.4345, "px left"=631.39185, "py left"=376.6227, "py right"=364.3492, "px right"=651.2822, "fy right"=921.49005, "fx right"=923.5849, "k left"=[0.13533829, -0.40519878, 0.0008784002, -0.0011180333, 0.3588802], "k right"=[0.12740475, -0.39763576, 0.00037952562, -0.0022863527, 0.35284942], "RLeft"=[0.9999986, 0.0009555143, -0.001359244, -0.0009574645, 0.9999985, -0.001434832, 0.001357871, 0.0014361315, 0.99999803], "Rright"=[0.99998456, -0.0019937593, -0.0051888847, 0.002001206, 0.99999696, 0.0014302958, 0.0051860176, -0.0014406577, 0.9999855], "uint8 reserved1"=[0, 0, 0, 0, 0, 0, 0, 0, 0, 0, 0, 0, 0, 0, 0, 0, 0, 0, 0, 0, 0, 0, 0, 0, 0, 0, 0, 0, 0, 0, 0, 0, 0, 0, 0, 0, 0, 0, 0, 0, 0, 0, 0, 0, 0, 0, 0, 0, 0, 0, 0, 0, 0, 0, 0, 0, 0, 0, 0, 0, 0, 0, 0, 0, 0, 0, 0, 0, 0, 0, 0, 0, 0, 0, 0, 0, 0, 0, 0, 0, 0, 0, 0, 0, 0, 0, 0, 0], "uint8 reserved2"=[0, 0, 0, 0, 0, 0, 0, 0, 0, 0, 0, 0, 0, 0, 0, 0, 0, 0, 0, 0, 0, 0, 0, 0, 0, 0, 0, 0, 0, 0, 0, 0, 0, 0, 0, 0, 0, 0, 0, 0, 0, 0, 0, 0, 0, 0, 0, 0, 0, 0, 0, 0, 0, 0, 0, 0, 0, 0, 0, 0, 0, 0, 0, 0], "1920x1080"=[1428.9095, 1428.9095, 951.85925, 556.0496], "1280x720"=[952.6064, 952.6064, 634.5728, 370.69974], "640x480"=[635.0709, 635.0709, 316.38187, 247.13316], "848x480"=[635.0709, 635.0709, 420.38187, 247.13316], "640x360"=[476.3032, 476.3032, 317.2864, 185.34987], "424x240"=[317.53546, 317.53546, 210.19093, 123.56658], "320x240"=[317.53546, 317.53546, 158.19093, 123.56658], "480x270"=[357.2274, 357.2274, 237.96481, 139.0124], "1280x800"=[1058.4515, 1058.4515, 633.9698, 411.8886], "960x540"=[714.4548, 714.4548, 475.92963, 278.0248], "Reserved1"=[714.4548, 714.4548, 475.92963, 278.0248], "Reserved 2"=[714.4548, 714.4548, 475.92963, 278.0248]} ("Calibration table"), "version"=w30, "table type"=w63, "table size"=w62, "full version"=w61, "crc32"=w60, "baseline"=w33, "model"=w32, "fx left"=w45, "fy left"=w44, "px left"=w43, "py left"=w42, "py right"=w41, "px right"=w40, "fy right"=w38, "fx right"=w39, "k left"=w37, "k right"=w36, "RLeft"=w35, "Rright"=w34, "uint8 reserved1"=w59, "uint8 reserved2"=w18, "1920x1080"=w58, "1280x720"=w31, "640x480"=w57, "848x480"=w56, "640x360"=w55, "424x240"=w54, "320x240"=w53, "480x270"=w52, "1280x800"=w51, "960x540"=w50, "Reserved1"=w21, "Reserved 2"=w20) -> (w23:T2)
  "Calibration table" <- w23
  n108 = Array Size(array=w18) -> (size(s)=→"size(s) 2":i32)
  n109 = Bundle By Name(cluster=T1 {"fx"=0.0, "fy"=0.0, "px"=0.0, "py"=0.0, "k left"=[], "fx2"=0.0, "fy2"=0.0, "py2"=0.0, "px2"=0.0, "k right"=[], "RLeft"=[0.999993, 0.0026725], "Rright"=[], "baseline"=0.0, "useBrownModel"=0, "1280x720"=[]} ("New Calibration Parameters"), "fx"=w45, "fy"=w44, "px"=w43, "py"=w42, "k left"=w37, "fx2"=w39, "fy2"=w38, "py2"=w41, "px2"=w40, "k right"=w36, "RLeft"=w35, "Rright"=w34, "baseline"=w33, "useBrownModel"=w32, "1280x720"=w31) -> (→"New Calibration Parameters":T1)
  n110 = disable-structure shown="Enabled" {
    disable-tunnel: w23 -> [w288 _]
    frame Enabled {
      w208 = u8[] [0]
      # "DS5CalibrationCoefficientsTable\n\n0-3  Command  0x15,0,0,0\n\n4-19\t Header\nuint16_t version;                       //!< Table version\n\tuint16_t tableType;                     //!< Table type\n\tuint32_t tableSize;                     //!< Table size \n\tuint32_t fullVersion;                   //!< Complete version of the table\n\tuint32_t crc32; \n\n20-   Table\n\n\tDS5CoeffsIntrinsics instrinsicsLeft;    //!< Intrinsics of the left camera\n   \tfloat fx;                               //!< Focal length in x axis, normalized by width\n   \tfloat fy;                               //!< Focal length in y axis, normalized by height\n\t   float px;                               //!< Principal point x axis coordinate, normalized by width\n\t   float py;                               //!< Principal point y axis coordinate, normalized by height\n\t   float k[5];                             //!< Distortion coefficients\n\tDS5CoeffsIntrinsics instrinsicsRight;   //!< Intrinsics of the right camera\n   \tfloat fx;                               //!< Focal length in x axis, normalized by width\n   \tfloat fy;                               //!< Focal length in y axis, normalized by height\n\t   float px;                               //!< Principal point x axis coordinate, normalized by width\n\t   float py;                               //!< Principal point y axis coordinate, normalized by height\n\t   float k[5];                             //!< Distortion coefficients\t\nfloat Rleft[9];                         //!< Inverse rotation of the left camera in rectified coordinate system\nfloat Rright[9];                        //!< Inverse rotation of the left camera in rectified coordinate system\n\tfloat B;                                //!< Baseline (maintains polarity)\n\tuint32_t useBrownModel;                 //!< Whether to use Brown or TYZX distrotion model (tangential distortion)\n\tuint8_t  reserved[88];                  //!< Reserved\n\n\n12x \n\tfloat rfx;                              //!< Rectified focal length in x axis\n\tfloat rfy;                              //!< Rectified focal length in y axis\n\tfloat rpx;                              //!< Rectified principal point x axis coordinate\n\tfloat rpy;                              //!< Rectified principal point y axis coordinate\n\n64x reserved"
      n111 = Unbundle By Name(w288) -> ("version"=w286:u16, "table type"=w284:u16, "table size"=w282:u32, "full version"=w277:u32, "crc32"=w275:u32, "baseline"=w236:sgl, "model"=w234:u32, "fx left"=w271:sgl, "fy left"=w269:sgl, "px left"=w268:sgl, "py left"=w267:sgl, "py right"=w244:sgl, "px right"=w245:sgl, "fy right"=w246:sgl, "fx right"=w247:sgl, "k left"=w257:sgl[], "k right"=w243:sgl[], "RLeft"=w241:sgl[], "Rright"=w240:sgl[], "uint8 reserved1"=w201:u8[], "uint8 reserved2"=w200:u8[], "1920x1080"=w230:sgl[], "1280x720"=w229:sgl[], "640x480"=w228:sgl[], "848x480"=w227:sgl[], "640x360"=w226:sgl[], "424x240"=w225:sgl[], "320x240"=w224:sgl[], "480x270"=w223:sgl[], "1280x800"=w222:sgl[], "960x540"=w221:sgl[], "Reserved1"=w204:sgl[], "Reserved 2"=w203:sgl[])
      n112 = for {
        tunnel: [w351] -> w258 mode=concatenating
        tunnel: w257 -> [w350] mode=indexing
        tunnel: w208 -> [w349]
        n113 = Type Cast(type=w349, x=w350) -> (*(type *) &x=w352:u8[])
        n114 = Reverse 1D Array(array=w352) -> (reversed array=w351:u8[])
      }
      n115 = Type Cast(type=w208, x=w234) -> (*(type *) &x=w235:u8[])
      n116 = for {
        tunnel: [w343] -> w239 mode=concatenating
        tunnel: w208 -> [w342]
        tunnel: w241 -> [w341] mode=indexing
        n117 = Type Cast(type=w342, x=w341) -> (*(type *) &x=w344:u8[])
        n118 = Reverse 1D Array(array=w344) -> (reversed array=w343:u8[])
      }
      n119 = Type Cast(type=w208, x=w236) -> (*(type *) &x=w237:u8[])
      n120 = for {
        tunnel: [w335] -> w220 mode=concatenating
        tunnel: w208 -> [w334]
        tunnel: w230 -> [w333] mode=indexing
        n121 = Type Cast(type=w334, x=w333) -> (*(type *) &x=w336:u8[])
        n122 = Reverse 1D Array(array=w336) -> (reversed array=w335:u8[])
      }
      n123 = for {
        tunnel: [w331] -> w219 mode=concatenating
        tunnel: w208 -> [w330]
        tunnel: w229 -> [w329] mode=indexing
        n124 = Type Cast(type=w330, x=w329) -> (*(type *) &x=w332:u8[])
        n125 = Reverse 1D Array(array=w332) -> (reversed array=w331:u8[])
      }
      n126 = for {
        tunnel: [w327] -> w218 mode=concatenating
        tunnel: w208 -> [w326]
        tunnel: w228 -> [w325] mode=indexing
        n127 = Type Cast(type=w326, x=w325) -> (*(type *) &x=w328:u8[])
        n128 = Reverse 1D Array(array=w328) -> (reversed array=w327:u8[])
      }
      n129 = for {
        tunnel: [w323] -> w217 mode=concatenating
        tunnel: w208 -> [w322]
        tunnel: w227 -> [w321] mode=indexing
        n130 = Type Cast(type=w322, x=w321) -> (*(type *) &x=w324:u8[])
        n131 = Reverse 1D Array(array=w324) -> (reversed array=w323:u8[])
      }
      n132 = for {
        tunnel: [w319] -> w216 mode=concatenating
        tunnel: w208 -> [w318]
        tunnel: w226 -> [w317] mode=indexing
        n133 = Type Cast(type=w318, x=w317) -> (*(type *) &x=w320:u8[])
        n134 = Reverse 1D Array(array=w320) -> (reversed array=w319:u8[])
      }
      n135 = for {
        tunnel: [w295] -> w207 mode=concatenating
        tunnel: w208 -> [w294]
        tunnel: w204 -> [w293] mode=indexing
        n136 = Type Cast(type=w294, x=w293) -> (*(type *) &x=w296:u8[])
        n137 = Reverse 1D Array(array=w296) -> (reversed array=w295:u8[])
      }
      n138 = for {
        tunnel: [w291] -> w206 mode=concatenating
        tunnel: w208 -> [w290]
        tunnel: w203 -> [w289] mode=indexing
        n139 = Type Cast(type=w290, x=w289) -> (*(type *) &x=w292:u8[])
        n140 = Reverse 1D Array(array=w292) -> (reversed array=w291:u8[])
      }
      n141 = Type Cast(type=w208, x=w284) -> (*(type *) &x=w285:u8[])
      n142 = Type Cast(type=w208, x=w277) -> (*(type *) &x=w278:u8[])
      n143 = Type Cast(type=w208, x=w271) -> (*(type *) &x=w272:u8[])
      n144 = Type Cast(type=w208, x=w269) -> (*(type *) &x=w266:u8[])
      n145 = Type Cast(type=w208, x=w268) -> (*(type *) &x=w265:u8[])
      n146 = Type Cast(type=w208, x=w267) -> (*(type *) &x=w264:u8[])
      n147 = Type Cast(type=w208, x=w282) -> (*(type *) &x=w283:u8[])
      n148 = Type Cast(type=w208, x=w275) -> (*(type *) &x=w274:u8[])
      n149 = Type Cast(type=w208, x=w286) -> (*(type *) &x=w287:u8[])
      n150 = Reverse 1D Array(array=w235) -> (reversed array=w232:u8[])
      n151 = Reverse 1D Array(array=w237) -> (reversed array=w233:u8[])
      n152 = Reverse 1D Array(array=w285) -> (reversed array=w280:u8[])
      n153 = Reverse 1D Array(array=w278) -> (reversed array=w276:u8[])
      n154 = Reverse 1D Array(array=w274) -> (reversed array=w273:u8[])
      n155 = Reverse 1D Array(array=w287) -> (reversed array=w281:u8[])
      n156 = Reverse 1D Array(array=w272) -> (reversed array=w270:u8[])
      n157 = Reverse 1D Array(array=w266) -> (reversed array=w263:u8[])
      n158 = Reverse 1D Array(array=w265) -> (reversed array=w262:u8[])
      n159 = Reverse 1D Array(array=w264) -> (reversed array=w261:u8[])
      n160 = Reverse 1D Array(array=w283) -> (reversed array=w279:u8[])
      n161 = Build Array (concatenate)(w270, w263, w262, w261, w258) -> (w259:u8[])
      n162 = Build Array (concatenate)(w233, w232, w201) -> (w231:u8[])
      n163 = Build Array (concatenate)(w281, w280, w279, w276, w273) -> (w260:u8[])
      n164 = for {
        tunnel: [w339] -> w238 mode=concatenating
        tunnel: w208 -> [w338]
        tunnel: w240 -> [w337] mode=indexing
        n165 = Type Cast(type=w338, x=w337) -> (*(type *) &x=w340:u8[])
        n166 = Reverse 1D Array(array=w340) -> (reversed array=w339:u8[])
      }
      n167 = for {
        tunnel: [w347] -> w256 mode=concatenating
        tunnel: w208 -> [w346]
        tunnel: w243 -> [w345] mode=indexing
        n168 = Type Cast(type=w346, x=w345) -> (*(type *) &x=w348:u8[])
        n169 = Reverse 1D Array(array=w348) -> (reversed array=w347:u8[])
      }
      n170 = Type Cast(type=w208, x=w247) -> (*(type *) &x=w248:u8[])
      n171 = Type Cast(type=w208, x=w246) -> (*(type *) &x=w250:u8[])
      n172 = Type Cast(type=w208, x=w245) -> (*(type *) &x=w251:u8[])
      n173 = Type Cast(type=w208, x=w244) -> (*(type *) &x=w252:u8[])
      n174 = for {
        tunnel: [w315] -> w215 mode=concatenating
        tunnel: w208 -> [w314]
        tunnel: w225 -> [w313] mode=indexing
        n175 = Type Cast(type=w314, x=w313) -> (*(type *) &x=w316:u8[])
        n176 = Reverse 1D Array(array=w316) -> (reversed array=w315:u8[])
      }
      n177 = for {
        tunnel: [w311] -> w214 mode=concatenating
        tunnel: w208 -> [w310]
        tunnel: w224 -> [w309] mode=indexing
        n178 = Type Cast(type=w310, x=w309) -> (*(type *) &x=w312:u8[])
        n179 = Reverse 1D Array(array=w312) -> (reversed array=w311:u8[])
      }
      n180 = for {
        tunnel: [w307] -> w213 mode=concatenating
        tunnel: w208 -> [w306]
        tunnel: w223 -> [w305] mode=indexing
        n181 = Type Cast(type=w306, x=w305) -> (*(type *) &x=w308:u8[])
        n182 = Reverse 1D Array(array=w308) -> (reversed array=w307:u8[])
      }
      n183 = for {
        tunnel: [w303] -> w212 mode=concatenating
        tunnel: w208 -> [w302]
        tunnel: w222 -> [w301] mode=indexing
        n184 = Type Cast(type=w302, x=w301) -> (*(type *) &x=w304:u8[])
        n185 = Reverse 1D Array(array=w304) -> (reversed array=w303:u8[])
      }
      n186 = for {
        tunnel: [w299] -> w211 mode=concatenating
        tunnel: w208 -> [w298]
        tunnel: w221 -> [w297] mode=indexing
        n187 = Type Cast(type=w298, x=w297) -> (*(type *) &x=w300:u8[])
        n188 = Reverse 1D Array(array=w300) -> (reversed array=w299:u8[])
      }
      n189 = Reverse 1D Array(array=w248) -> (reversed array=w249:u8[])
      n190 = Reverse 1D Array(array=w250) -> (reversed array=w253:u8[])
      n191 = Reverse 1D Array(array=w251) -> (reversed array=w254:u8[])
      n192 = Reverse 1D Array(array=w252) -> (reversed array=w255:u8[])
      n193 = Build Array (concatenate)(w249, w253, w254, w255, w256) -> (w242:u8[])
      n194 = Array Size(array=w200) -> (size(s)=→"size(s)":i32)
      n195 = Build Array (concatenate)(w220, w219, w218, w217, w216, w215, w214, w213, w212, w211, w207, w206) -> (w210:u8[])
      n196 = Build Array (concatenate)(w260, w259, w242, w239, w238, w231, w210, w200) -> (w205:u8[])
      "Output array" <- w205
      n197 = Array Size(array=w205) -> (size(s)=→"size":i32)
    }
    frame Disabled {
    }
  }
